vi "Split_8BitData.vi"(1 "x":u8 format="%.0x") -> (14 "hi(x)":u8 format="%x", 16 "lo(x)":u8 format="%.0x")   [LabVIEW 2023, in "HardwareAbstractionLayer_LVOOP.lvlib" / "CAN Application Protocols Lib.lvlib" / "STP Protocol.lvclass"]
uses:
  STP Protocol.lvclass
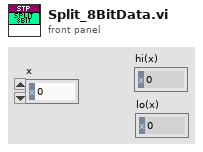
[diagram p1: front panel]
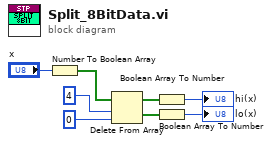
[diagram p0: block diagram]
diagram:
  n1 = Number To Boolean Array(number="x") -> (Boolean array=w7:bool[])
  n2 = Delete From Array(array=w7, length=4 ("dimension size"), index=0) -> (deleted portion=w3:bool[], array with subset deleted=w4:bool[])
  n3 = Boolean Array To Number(Boolean array=w4) -> (number=→"hi(x)":u32)
  n4 = Boolean Array To Number(Boolean array=w3) -> (number=→"lo(x)":u32)
